vi "Get-Set order.vi"(8 "error in":errorcluster, 10 "Approved order in":T1, 11 "Get-Set":T2) -> (0 "error out":errorcluster, 3 "Approved order out":T1)   [LabVIEW 2015]
doc: "Get or set order for state after start pressing."
uses:
  Controls/Approved order.ctl
  Controls/Get-Set.ctl
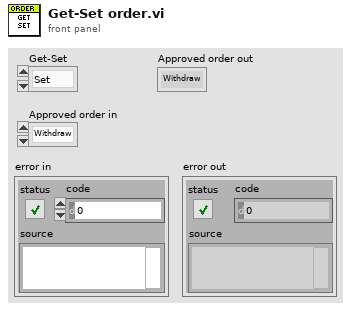
[diagram p1: front panel]
types:
  T1 = typedef "Approved order.ctl" = enum16{"Withdraw", "Balance", "Deposit", "Verify"}
  T2 = typedef "Get-Set.ctl" = enum16{"Set", "Get"}
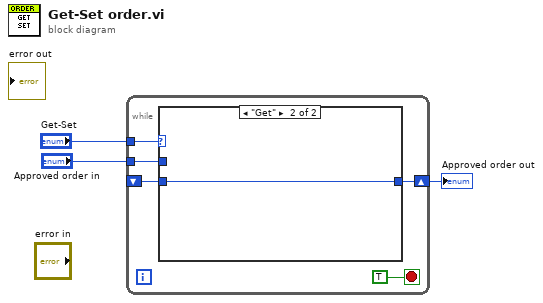
[diagram p0: block diagram]
diagram:
  n1 = while {
    tunnel: "Get-Set" -> [w7]
    shift-right: [w6] -> w3
    shift-left: _ -> [w4]
    tunnel: "Approved order in" -> [w5]
    stop <- TRUE stop-if-true
    n2 = case shown="\"Get\"" w7 {
      tunnel: [w9 w10] -> w6
      tunnel: w5 -> [w9 _]
      tunnel: w4 -> [_ w10]
      frame "Set", Default {
      }
      frame "Get" {
      }
    }
  }
  "Approved order out" <- w3
